vi "test_Packet_SimpleTrackedTarget.vi"(8 "error in (no error)":errorcluster) -> (0 "error out":errorcluster, 3 "Test Passed":bool)   [LabVIEW 2019]
uses:
  PhotonVisionLib/PhotonVisionLib.lvlib
  <vilib>/Rock Robotics/WPI/ThirdParty/JAS_Junk/TrajLib/Trajectory_Library.lvlib
  PhotonVisionLib/TypeDef/TargetCornerType.ctl
  PhotonVisionLib/TypeDef/PhotonTrackedTargetType.ctl
  <vilib>/Rock Robotics/WPI/ThirdParty/JAS_Junk/TrajLib/TypeDef/TRANSLATION3D.ctl
  <vilib>/Rock Robotics/WPI/ThirdParty/JAS_Junk/TrajLib/TypeDef/QUATERNION.ctl
  <vilib>/Rock Robotics/WPI/ThirdParty/JAS_Junk/TrajLib/TypeDef/ROTATION3D.ctl
  <vilib>/Rock Robotics/WPI/ThirdParty/JAS_Junk/TrajLib/TypeDef/TRANSFORM3D.ctl
panel:
  out "TrackedTarget 2":T1={"Yaw"=0.0, "Pitch"=0.0, "Area"=0.0, "Skew"=0.0, "MinAreaRectCorners"=[], "BestCameraToTarget"={"TRANSLATION3D"={"X"=0.0, "Y"=0.0, "Z"=0.0}, "ROTATION3D"={"Q_quaternion"={"R"=1.0, "V"=[0.0, 0.0, 0.0]}}, "XF"=FALSE}, "FiiducialId"=0, "AltCameraToTarget"={"TRANSLATION3D"={"X"=0.0, "Y"=0.0, "Z"=0.0}, "ROTATION3D"={"Q_quaternion"={"R"=1.0, "V"=[0.0, 0.0, 0.0]}}, "XF"=FALSE}, "PoseAmbiguity"=0.0, "DetectedCorners"=[]} {"AltCameraToTarget"."TRANSLATION3D"."Z" format="%14.3f"; "AltCameraToTarget"."TRANSLATION3D"."Y" format="%14.3f"; "AltCameraToTarget"."TRANSLATION3D"."X" format="%14.3f"; "BestCameraToTarget"."TRANSLATION3D"."Z" format="%14.3f"; "BestCameraToTarget"."TRANSLATION3D"."Y" format="%14.3f"; "BestCameraToTarget"."TRANSLATION3D"."X" format="%14.3f"}
  out "TrackedTarget":T1={"Yaw"=0.0, "Pitch"=0.0, "Area"=0.0, "Skew"=0.0, "MinAreaRectCorners"=[], "BestCameraToTarget"={"TRANSLATION3D"={"X"=0.0, "Y"=0.0, "Z"=0.0}, "ROTATION3D"={"Q_quaternion"={"R"=1.0, "V"=[0.0, 0.0, 0.0]}}, "XF"=FALSE}, "FiiducialId"=0, "AltCameraToTarget"={"TRANSLATION3D"={"X"=0.0, "Y"=0.0, "Z"=0.0}, "ROTATION3D"={"Q_quaternion"={"R"=1.0, "V"=[0.0, 0.0, 0.0]}}, "XF"=FALSE}, "PoseAmbiguity"=0.0, "DetectedCorners"=[]} {"AltCameraToTarget"."TRANSLATION3D"."Z" format="%14.3f"; "AltCameraToTarget"."TRANSLATION3D"."Y" format="%14.3f"; "AltCameraToTarget"."TRANSLATION3D"."X" format="%14.3f"; "BestCameraToTarget"."TRANSLATION3D"."Z" format="%14.3f"; "BestCameraToTarget"."TRANSLATION3D"."Y" format="%14.3f"; "BestCameraToTarget"."TRANSLATION3D"."X" format="%14.3f"}
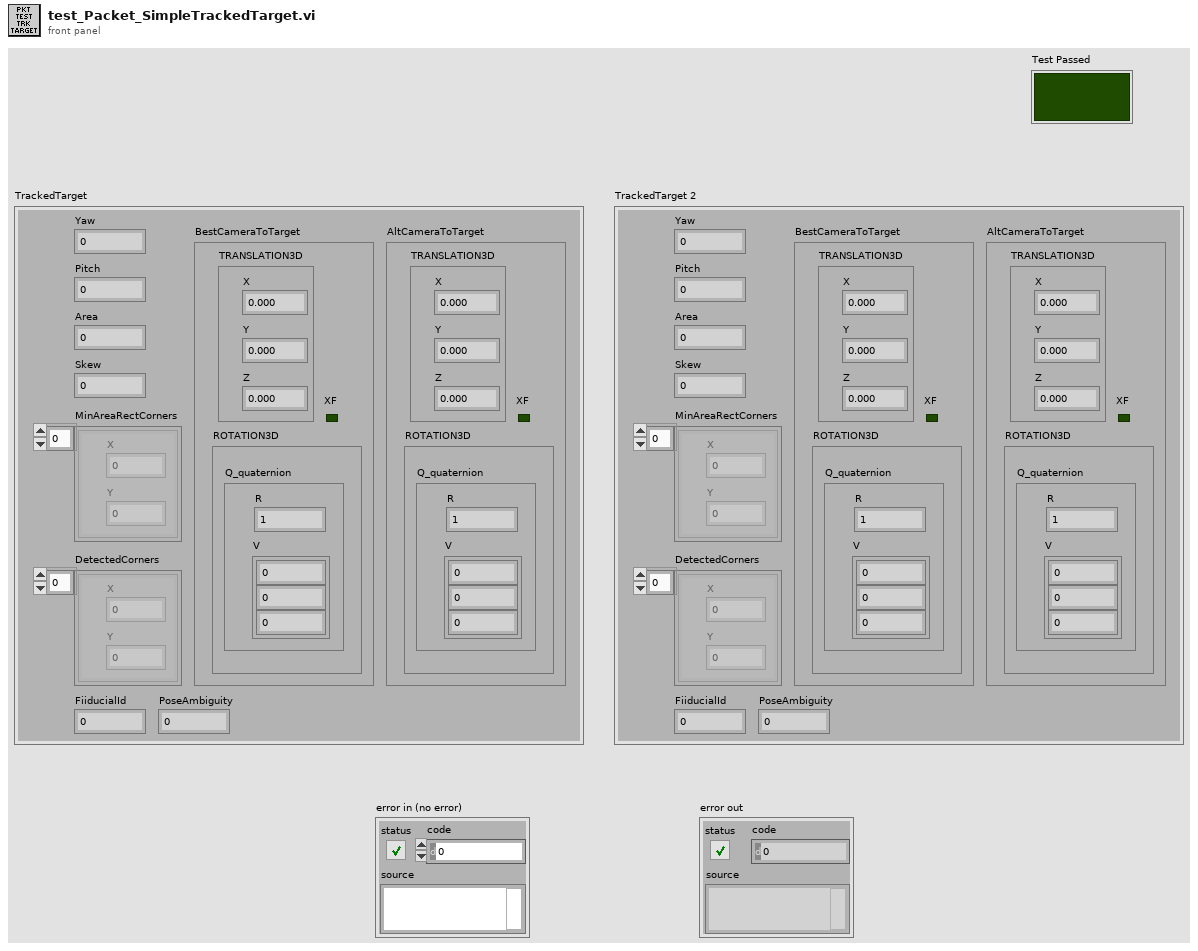
[diagram p1: front panel]
types:
  T1 = typedef "PhotonVisionLib.lvlib/PhotonTrackedTargetType.ctl" = cluster{"Yaw":dbl, "Pitch":dbl, "Area":dbl, "Skew":dbl, "MinAreaRectCorners":T2[], "BestCameraToTarget":T3, "FiiducialId":i32, "AltCameraToTarget":T3, "PoseAmbiguity":dbl, "DetectedCorners":T2[]}
  T2 = typedef "PhotonVisionLib.lvlib/TargetCornerType.ctl" = cluster{"X":dbl, "Y":dbl}
  T3 = typedef "Trajectory_Library.lvlib/TRANSFORM3D.ctl" = cluster{"TRANSLATION3D":T4, "ROTATION3D":T5, "XF":bool}
  T4 = typedef "Trajectory_Library.lvlib/TRANSLATION3D.ctl" = cluster{"X":dbl, "Y":dbl, "Z":dbl}
  T5 = typedef "Trajectory_Library.lvlib/ROTATION3D.ctl" = cluster{"Q_quaternion":T6}
  T6 = typedef "Trajectory_Library.lvlib/QUATERNION.ctl" = cluster{"R":dbl, "V":dbl[]}
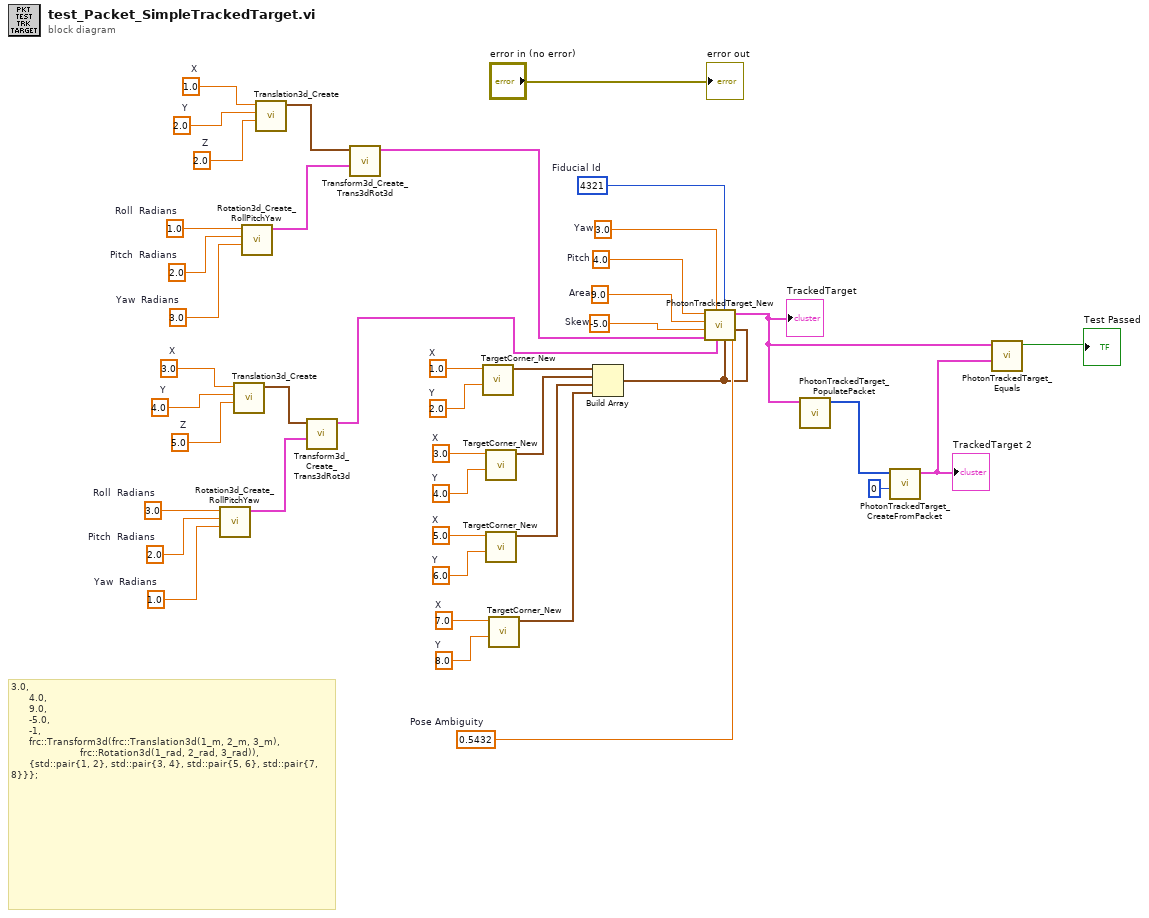
[diagram p0: block diagram]
diagram:
  w6 = 3.0  # Roll  Radians
  w5 = 2.0  # Pitch  Radians
  w4 = 1.0  # Yaw  Radians
  w8 = 3.0  # X
  w9 = 4.0  # Y
  w10 = 5.0  # Z
  w15 = 1.0  # Roll  Radians
  w14 = 2.0  # Pitch  Radians
  w13 = 3.0  # Yaw  Radians
  w17 = 1.0  # X
  w18 = 2.0  # Y
  w19 = 2.0  # Z
  w20 = 0.5432  # Pose Ambiguity
  w21 = 4321  # Fiducial Id
  w27 = 4.0  # Pitch
  w28 = 9.0  # Area
  w29 = -5.0  # Skew
  w30 = 3.0  # Yaw
  w35 = 7.0  # X
  w36 = 8.0  # Y
  w37 = 5.0  # X
  w38 = 6.0  # Y
  w39 = 3.0  # X
  w40 = 4.0  # Y
  w41 = 1.0  # X
  w42 = 2.0  # Y
  # "3.0,\n      4.0,\n      9.0,\n      -5.0,\n      -1,\n      frc::Transform3d(frc::Translation3d(1_m, 2_m, 3_m),\n                       frc::Rotation3d(1_rad, 2_rad, 3_rad)),\n      {std::pair{1, 2}, std::pair{3, 4}, std::pair{5, 6}, std::pair{7, 8}}};"
  n1 = call <vilib>:"Rotation3d_Create_RollPitchYaw.vi"("Yaw"=w4, "Pitch"=w5, "Roll"=w6) -> ("Rotation3d"=w3:T5)  [unwired: 8 in]
  n2 = call <vilib>:"Translation3d_Create.vi"("Z"=w10, "Y"=w9, "X"=w8) -> ("TRANSLATION3D"=w7:T4)  [unwired: 8 in]
  n3 = call <vilib>:"Rotation3d_Create_RollPitchYaw.vi"("Yaw"=w13, "Pitch"=w14, "Roll"=w15) -> ("Rotation3d"=w12:T5)  [unwired: 8 in]
  n4 = call <vilib>:"Translation3d_Create.vi"("Z"=w19, "Y"=w18, "X"=w17) -> ("TRANSLATION3D"=w16:T4)  [unwired: 8 in]
  n5 = call <vilib>:"Transform3d_Create_Trans3dRot3d.vi"("Rotation3d"=w3, "Translation3d"=w7) -> ("Transform3d"=w2:T3)  [unwired: 9 in]
  n6 = call <vilib>:"Transform3d_Create_Trans3dRot3d.vi"("Rotation3d"=w12, "Translation3d"=w16) -> ("Transform3d"=w11:T3)  [unwired: 9 in]
  n7 = call "TargetCorner_New.vi"("Y"=w42, "X"=w41) -> ("TargetCorner"=w34:T2)  [unwired: 9 in]
  n8 = call "TargetCorner_New.vi"("Y"=w40, "X"=w39) -> ("TargetCorner"=w33:T2)  [unwired: 9 in]
  n9 = call "TargetCorner_New.vi"("Y"=w38, "X"=w37) -> ("TargetCorner"=w32:T2)  [unwired: 9 in]
  n10 = call "TargetCorner_New.vi"("Y"=w36, "X"=w35) -> ("TargetCorner"=w31:T2)  [unwired: 9 in]
  n11 = Build Array(w34, w33, w32, w31) -> (w1:T2[])
  n12 = call "PhotonTrackedTarget_New.vi"("Pose Ambiguity"=w20, "DetectedCorners"=w1, "MinAreaRectCorners"=w1, "Fiducial Id"=w21, "AltCameraToTarget"=w2, "Yaw"=w30, "BestCameraToTarget"=w11, "Skew"=w29, "Area"=w28, "Pitch"=w27) -> ("TrackedTarget"=w24:T1)  [unwired: 1 in]
  "TrackedTarget" <- w24
  n13 = call "PhotonTrackedTarget_PopulatePacket.vi"("TrackedTarget"=w24) -> ("RawData Out"=w26:u8[])  [unwired: 10 in]
  n14 = call "PhotonTrackedTarget_CreateFromPacket.vi"("StartByte"=0, "RawData"=w26) -> ("TrackedTarget"=w23:T1)  [unwired: 8 in, 1 out]
  "TrackedTarget 2" <- w23
  n15 = call "PhotonTrackedTarget_Equals.vi"("Other TrackedTarget"=w23, "TrackedTarget"=w24) -> ("Equals"=→"Test Passed":bool)  [unwired: 9 in]
  "error out" <- "error in (no error)"
